vi "Dashboard Main.vi"() -> ()   [LabVIEW 2015]
uses:
  <vilib>/vision/Image Controls.llb/IMAQ Image.ctl
  <vilib>/Utility/miscctls.llb/LVRowAndColumnTypeDef.ctl
  <vilib>/event_ctls.llb/eventvkey.ctl
  <vilib>/Rock Robotics/WPI/Dashboard/WPI_DashboardLogging Global.vi
  <vilib>/Rock Robotics/Network Tables/NT Read Numeric Array.vi
  <vilib>/Rock Robotics/Network Tables/NT Read Boolean.vi
  <vilib>/Rock Robotics/Network Tables/NT Read Raw.vi
  <vilib>/Rock Robotics/Network Tables/NT Write Boolean.vi
  <vilib>/Utility/config.llb/Write Key (String).vi
  <vilib>/Utility/config.llb/Write Key (I32).vi
  <vilib>/Utility/config.llb/NI_LVConfig.lvlib
panel:
  in  "TCP":refnum<k5>
  in  "Rec Mode":enum32{"Stop", "Record", "Playback"}(radio)
  in  "Vision":u16(ring) items=["Camera Off", "USB Camera SW", "USB Camera HW", "IP Camera"]
  out "Camera IP":string
  out "Image Message":string="Timeout in Camera Communications"
  in  "Dashboard Tab":T1(tab)
  in  "CDF":bool
  in  "Position":i8
  in  "Power":i8(slide) scale=0.0..100.0
  in  "Select Auto":string(combo)
  out "NT Connection":bool
  in  "Camera Settings":T2={"Frame Rate"=30, "Compression"=30, "Size"=1} {"Frame Rate" scale=1.0..30.0; "Size" items=["640x480", "320x240", "160x120"]}
  out "MotorChart R":cluster{"Numeric":dbl, "Numeric":dbl}(graph)
  out "MotorChart L":T3(graph)
  out "MotorSliders R":cluster{"MotorSlide1":dbl, "MotorSlide2":dbl} {"MotorSlide2" scale=-1.0..1.0 scale format="%#_2e"; "MotorSlide1" scale=-1.0..1.0 scale format="%#_2e"}
  out "MotorSliders L":T4 {"MotorSlide4 2" scale=0.0..14.0 scale format="%#_2e"; "MotorSlide2" scale=-1.0..1.0 scale format="%#_2e"; "MotorSlide1" scale=-1.0..1.0 scale format="%#_2e"}
  out "JS1 Z":dbl(slide) scale=-1.0..1.0 scale format="%#_2e"
  out "JS1 Graph":cluster{"X":dbl, "Y":dbl}[](graph)
  out "JS1 Buttons":T5
  out "JS2 Z":dbl(slide) scale=-1.0..1.0 scale format="%#_2e"
  out "JS2 Graph":cluster{"X":dbl, "Y":dbl}[](graph)
  out "JS2 Buttons":T5
  out "Mode":T6(ring)=enum."Auto Disabled"
  in  "DB Camera Config":bool
  out "fps":dbl format="%#.1g"
  out "Mbps":dbl format="%#.1g"
  out "Mbps LED":bool
  in  "DB/String 9":string
  in  "DB/String 8":string
  in  "DB/String 7":string
  in  "DB/String 6":string
  in  "DB/String 5":string
  in  "DB/String 4":string
  in  "DB/String 3":string
  in  "DB/String 2":string
  in  "DB/String 1":string
  in  "DB/String 0":string
  in  "DB/Slider 0":dbl(slide) scale=0.0..5.0
  in  "DB/Slider 1":dbl(slide) scale=0.0..5.0
  in  "DB/Slider 2":dbl(slide) scale=0.0..5.0
  in  "DB/Slider 3":dbl(slide) scale=0.0..5.0
  out "DB/LED 3":bool
  out "DB/LED 2":bool
  out "DB/LED 1":bool
  out "DB/LED 0":bool
  in  "DB/Button 3":bool
  in  "DB/Button 2":bool
  in  "DB/Button 1":bool
  in  "DB/Button 0":bool caption="New Name"
  out "Masked Image":T7
  out "T3 Visible":bool
  out "T2 Visible":bool
  out "T1 Visible":bool
  out "Right":dbl(slide) scale=-1.0..1.0
  out "Left":dbl(slide) scale=-1.0..1.0
  out "T3 Y":dbl
  out "T3 X":dbl
  out "T2 Y":dbl
  out "T2 X":dbl
  out "TI Y":dbl
  out "T1 X":dbl
  out "T3 Dist":dbl
  out "T2 Dist":dbl
  out "T1 Dist":dbl
  out "Encoder 2 Dist":dbl
  out "Encoder 1 Dist":dbl
  out "Encoder 2 Dir":bool
  out "Encoder 1 Dir":bool
  in  "Test Slider":dbl(slide) scale=0.0..100.0 scale format="%#_3g"
  in  "On/Off":bool caption="Solenoid"
  in  "Test Name":u16(ring) items=["Select the test to run..."]
  in  "Test Tree":string(tree)
  in  "Motor":cluster{"Value":dbl, "Enable":bool} {"Value" scale=-1.0..1.0 scale format="%#_3g"}
  out "Progress":T8 {"Test Progress" scale=0.0..100.0}
  in  "Rev/Fwd":cluster{"Forward":bool, "Reverse":bool}
  in  "Test Ring":u16(ring) items=["Monochrome", "Color"]
  out "Cmd Status":string
  in  "Execute Command":bool
  in  "Command Params":string[][](table)
  in  "Command Selection":i32(listbox)
  in  "CheckList":i32(listbox)
  out "Tree":string(tree)
  out "Camera Image":T7(plugin-control)
  out "Background":bool
  # "Left"
  # "Front"
  # "Right"
  # "Battery"
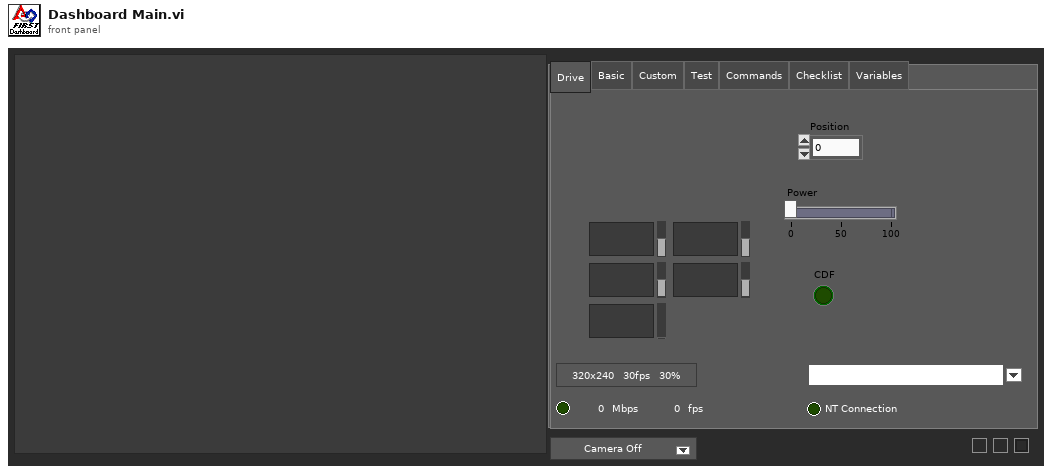
[diagram p1: front panel]
types:
  T1 = enum32{"Drive", "Basic", "Custom", "Test", "Commands", "Checklist", "Variables"}
  T2 = cluster{"Frame Rate":i32, "Compression":i32, "Size":u16}
  T3 = cluster{"Numeric":dbl, "Numeric":dbl, "Battery V":dbl}
  T4 = cluster{"MotorSlide1":dbl, "MotorSlide2":dbl, "MotorSlide4 2":dbl}
  T5 = cluster{bool, bool, bool, bool, bool, bool, bool, bool, bool, bool, bool, bool}
  T6 = enum8{"Tele-Op Disabled", "Tele-Op Enabled", "Auto Disabled", "Auto Enabled", "Test Disabled", "Test Enabled", "Disconnected", "No Code", "E-Stop"}
  T7 = typedef "IMAQ Image.ctl" = refnum<image>
  T8 = cluster{"Test Progress":u8, "Test Progress Text":string}
  T9 = cluster{"IDs":cluster{"RPC field ID":u16, "Unique ID":u16}, "String":string}
  T10 = enum32{"Drive", "Basic", "Custom", "Test", "Checklist", "Variables"}
  T11 = typedef "Image Type" = u32
  T12 = cluster{"Camera Image":refnum<vi>, "Dashboard Tab":refnum<vi>, "Background":refnum<vi>, "Vision":refnum<vi>, "Rec Mode":refnum<vi>, "Test Slider":refnum<vi>, "On/Off ":refnum<vi>, "Test Ring":refnum<vi>, "Rev/Fwd":refnum<vi>, "Test Name":refnum<vi>, "Motor":refnum<vi>, "Progress":refnum<vi>, "CheckList":refnum<vi>, "Tree":refnum<vi>, "Test Tree":refnum<vi>, "Command Params":refnum<vi>, "Command Selection":refnum<vi>, "Execute Command":refnum<vi>, "Cmd Status":refnum<vi>}
  T13 = cluster{"Error Strings":string, "Disable Counts":cluster{u16, u16}, "Rail Faults":cluster{u16, u16, u16}, "Robot IP":string, "DB Mode":u8, "Event Info":cluster{"Name":string, "Type":u8, "Number":u16, "Replay":u8}, "Camera Addr":string}
  T14 = cluster{"Storage":cluster{"Disk Free":u64, "RAM Block":u32, "RAM free":u32}, "CPU Utilization":cluster{"CPU % ISR":sgl, "CPU % Time Crit":sgl, "CPU % Timed Str":sgl, "CPU % High":sgl, "CPU % Above":sgl, "CPU % Normal":sgl, "CPU % Low":sgl}, "CAN":cluster{"% Bus Utilization":sgl, "Bus Off Cnt":u32, "TX_FIFO Full Cnt":u32, "Receive Error Cnt":u8, "Transmit Error Cnt":u8}, "HID":cluster{"HID Outputs":u32, "Rumble Low":u16, "Rumble High":u16}[]}
  T15 = cluster{"Status bits":cluster{"Test Mode":bool, "Autonomous":bool, "Enabled":bool, "Code Start":bool, "Brownout":bool, "Reserved 2":bool, "Reserved 3":bool, "E-Stop":bool}, "Code Trace":cluster{"Disabled":bool, "TeleOp":bool, "Auto":bool, "Test":bool}, "Controller Type":enum16{"unknown", "cRIO", "roboRio"}, "Code?":enum16{"unknown", "noCode", "code"}, "Battery V":dbl}
  T16 = cluster{"Control Bits":cluster{"TestMode":bool, "Autonomous":bool, "Enabled":bool, "FMS Present":bool, bool, bool, bool, "E-Stop":bool}, "Team Station ":u8, "Countdown":sgl, "Joystick Values":cluster{"Axes":dbl[], "Buttons":bool[], "POVs":i16[]}[]}
  T17 = cluster{"Axes":dbl[], "Buttons":bool[], "POVs":i16[]}[]
  T18 = cluster{"Axes":dbl[], "Buttons":bool[], "POVs":i16[]}
  T19 = cluster{"Buttons[0]":bool, "Buttons[1]":bool, "Buttons[2]":bool, "Buttons[3]":bool, "Buttons[4]":bool, "Buttons[5]":bool, "Buttons[6]":bool, "Buttons[7]":bool, "Buttons[8]":bool, "Buttons[9]":bool, "Buttons[10]":bool, "Buttons[11]":bool}
  T20 = typedef "NI_LVConfig.lvlib/Config Data RefNum.ctl" = refnum<k1>
  T21 = cluster{"Operation":enum16{"Update", "Clear"}, "Color Box":u32}[]
  T22 = typedef "eventvkey.ctl" = enum16{"ASCII", "Enter", "Return", "Shift", "Ctrl", "Alt", "Cmd", "Opt", "Caps", "NumLock", "Clear", "Break", "Up", "Down", "Left", "Right", "Insert", "Delete", "Home", "End", "PageUp", "PageDown", "Escape", "Help", "Pause", "ScrollLock", "F1", "F2", "F3", "F4", "F5", "F6", "F7", "F8", "F9", "F10", "F11", "F12", "F13", "F14", "F15", "F16", "F17", "F18", "F19", "F20", "F21", "F22", "F23", "F24", "Play", "VolumeUp", "VolumeDown", "Mute", "Two Byte Char"}
  T23 = cluster{"Image Size":bool, "Image Type":bool, "Pixel Value":bool, "ROI Information":bool, "Zoom Factor":bool}
  T24 = enum8{"Enabled", "Disabled", "Disabled and Grayed Out"}
  T25 = cluster{"Operation":enum16{"Update", "Clear"}, "Color Box":u32}
  T26 = typedef "LVRowAndColumnTypeDef.ctl" = cluster{"Row":i32, "Column":i32}
  T27 = cluster{"Shift":bool, "Ctrl":bool, "Alt":bool, "Cmd":bool, "Opt":bool}
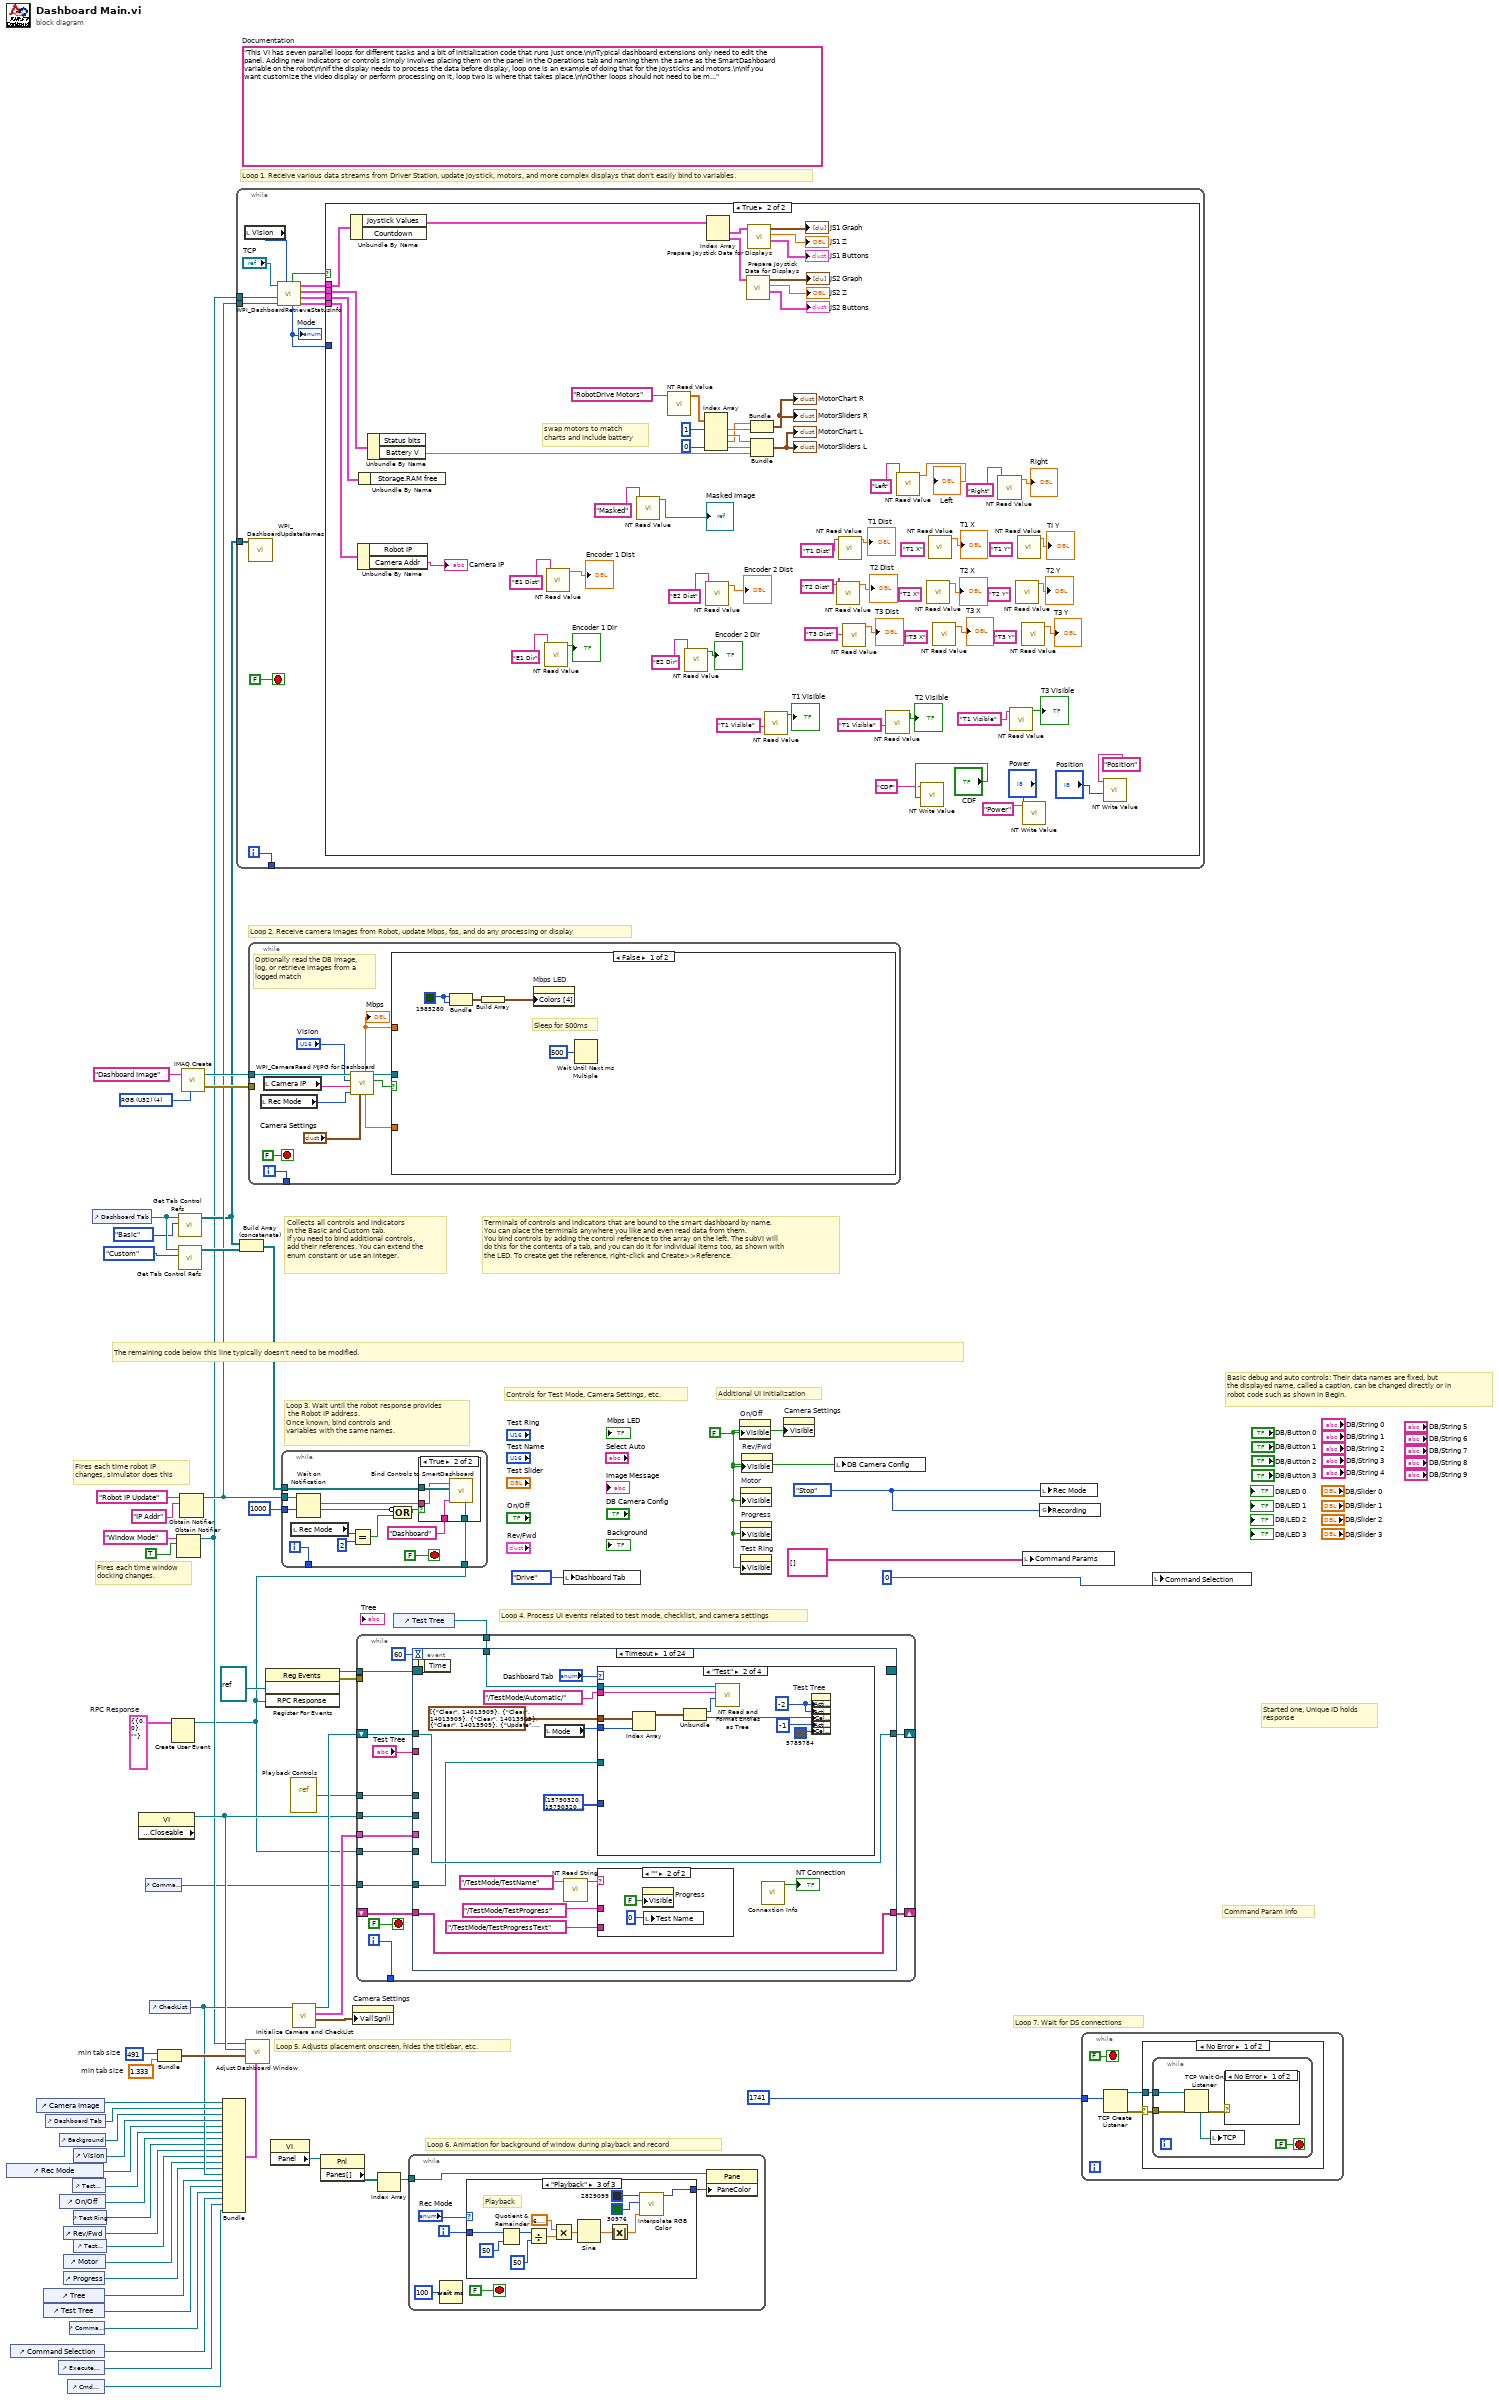
[diagram p0: block diagram]
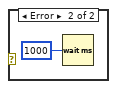
[diagram p2: hidden frame]
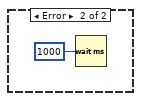
[diagram p3: hidden frame]
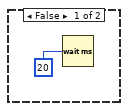
[diagram p4: hidden frame]
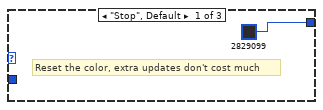
[diagram p5: hidden frame]
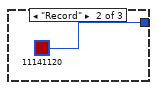
[diagram p6: hidden frame]
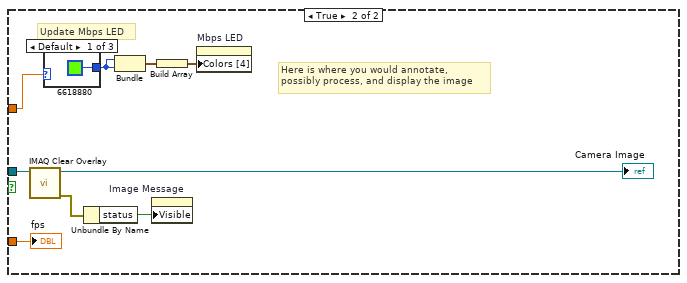
[diagram p8: hidden frame]
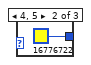
[diagram p9: hidden frame]
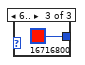
[diagram p10: hidden frame]
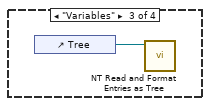
[diagram p12: hidden frame]
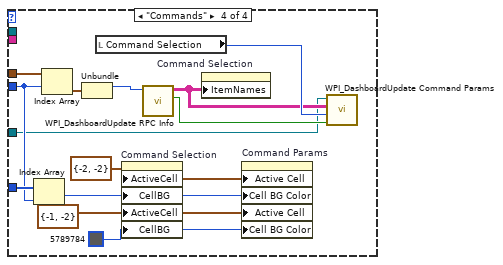
[diagram p13: hidden frame]
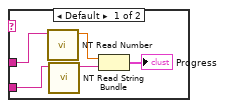
[diagram p14: hidden frame]
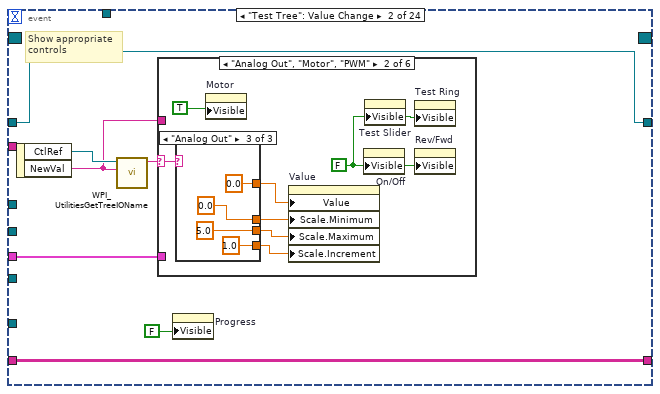
[diagram p15: hidden frame]
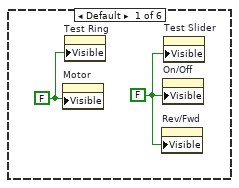
[diagram p16: hidden frame]
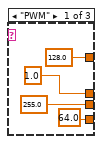
[diagram p17: hidden frame]
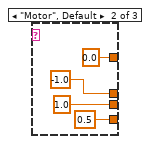
[diagram p18: hidden frame]
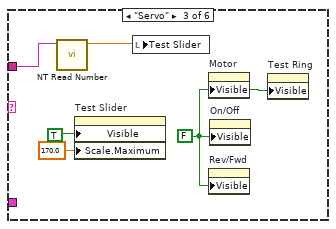
[diagram p19: hidden frame]
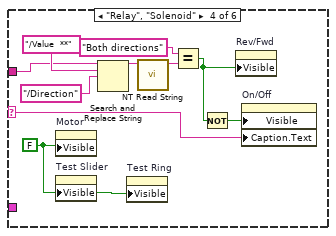
[diagram p20: hidden frame]
diagram:
  w7 = T9 {"IDs"={"RPC field ID"=0, "Unique ID"=0}, "String"=""}  # RPC Response
  w33 = 491  # min tab size
  w32 = 1.333  # min tab size
  w41 = enum32{"Stop", "Record", "Playback"}."Stop" ("Rec Mode")
  w15 = FALSE ("Visible")
  (unwired) "This VI has seven parallel loops for different tasks and a bit of initialization code that runs just once.\n\nTypical dashboard extensions only need to edit the panel. Adding new indicators or controls simply involves placing them on the panel in the Operations tab and naming them the same as the SmartDashboard variable on the robot\n\nIf the display needs to process the data before display, loop one is an example of doing that for the joysticks and motors.\n\nIf you want customize the video display or perform processing on it, loop two is where that takes place.\n\nOther loops should not need to be modified. They are pretty standard, and document the task they perform."  # Documentation
  w61 = T11 4 items=["Grayscale (U8)", "Grayscale (I16)", "Grayscale (SGL)", "Complex (CSG)", "RGB (U32)", "HSL (U32)", "RGB (U64)"] ("Image Type")
  # "Command Param Info"
  # "Started one, Unique ID holds\nresponse"
  # "Loop 7. Wait for DS connections"
  # "Basic debug and auto controls: Their data names are fixed, but\nthe displayed name, called a caption, can be changed directly or in\nrobot code such as shown in Begin."
  # "Controls for Test Mode, Camera Settings, etc."
  # "Additional UI Initialization"
  # "Loop 6. Animation for background of window during playback and record"
  # "Fires each time robot IP\nchanges, simulator does this"
  # "Fires each time window\ndocking changes."
  # "Collects all controls and indicators\nin the Basic and Custom tab.\nIf you need to bind additional controls,\nadd their references. You can extend the\nenum constant or use an integer."
  # "The remaining code below this line typically doesn't need to be modified."
  # "Loop 4. Process UI events related to test mode, checklist, and camera settings"
  # "Terminals of controls and indicators that are bound to the smart dashboard by name.\nYou can place the terminals anywhere you like and even read data from them.\nYou bind controls by adding the control reference to the array on the left. The subVI will\ndo this for the contents of a tab, and you can do it for individual items too, as shown with\nthe LED. To create get the reference, right-click and Create>>Reference."
  # "Loop 3. Wait until the robot response provides\n the Robot IP address.\nOnce known, bind controls and\nvariables with the same names."
  # "Loop 5. Adjusts placement onscreen, hides the titlebar, etc."
  # "Loop 1. Receive various data streams from Driver Station, update joystick, motors, and more complex displays that don't easily bind to variables."
  # "Loop 2. Receive camera images from Robot, update Mbps, fps, and do any processing or display"
  n1 = control-ref of="Rec Mode"() -> (w21:refnum<vi>)
  n2 = control-ref of="Command Selection"() -> (w6:refnum<vi>)
  n3 = control-ref of="Camera Image"() -> (w36:refnum<vi>)
  n4 = control-ref of="Tree"() -> (w25:refnum<vi>)
  n5 = control-ref of="Test Tree"() -> (w24:refnum<vi>)
  n6 = control-ref of="Dashboard Tab"() -> (w35:refnum<vi>)
  n7 = control-ref of="Execute Command"() -> (w8:refnum<vi>)
  n8 = control-ref of="Background"() -> (w30:refnum<vi>)
  n9 = control-ref of="On/Off"() -> (w19:refnum<vi>)
  n10 = control-ref of="Progress"() -> (w16:refnum<vi>)
  n11 = control-ref of="Rev/Fwd"() -> (w17:refnum<vi>)
  n12 = control-ref of="Motor"() -> (w22:refnum<vi>)
  n13 = control-ref of="Cmd Status"() -> (w2:refnum<vi>)
  n14 = control-ref of="Command Params"() -> (w9:refnum<vi>)
  n15 = control-ref of="Test Slider"() -> (w20:refnum<vi>)
  n16 = control-ref of="Vision"() -> (w34:refnum<vi>)
  n17 = control-ref of="Test Ring"() -> (w18:refnum<vi>)
  n18 = control-ref of="Test Name"() -> (w23:refnum<vi>)
  n19 = control-ref of="Dashboard Tab"() -> (w39:refnum<vi>)
  n20 = property class="VI" props=["Front Panel.Closeable"]() -> (reference out=w40:refnum<vi>)  [unwired: 2 in, 2 out]
  n21 = control-ref of="Command Params"() -> (w1:refnum<vi>)
  n22 = control-ref of="CheckList"() -> (w26:refnum<vi>)
  n23 = Bundle("min tab size"=w33, "min tab size"=w32) -> (w31:cluster{"min tab size":i32, "min tab size":dbl})  [unwired: 1 in]
  n24 = Create User Event(user event datatype=w7) -> (user event=w3:refnum<user-event>)  [unwired: 1 in, 1 out]
  n25 = Obtain Notifier(name (unnamed)="Window Mode", notification data type=TRUE) -> (notifier out=w12:refnum<notifier>)  [unwired: 2 in, 2 out]
  n26 = call <vilib>:"Get Tab Control Refs.vi"("Page Index"=T10."Basic" ("Dashboard Tab"), "TabControl in"=w39) -> ("ControlsOnPage"=w13:refnum<vi>[])  [unwired: 9 in]
  n27 = call <vilib>:"Get Tab Control Refs.vi"("Page Index"=T10."Custom" ("Dashboard Tab"), "TabControl in"=w39) -> ("ControlsOnPage"=w38:refnum<vi>[])  [unwired: 9 in]
  n28 = Obtain Notifier(name (unnamed)="Robot IP Update", notification data type="IP Addr" ("name (unnamed)")) -> (notifier out=w14:refnum<notifier>)  [unwired: 2 in, 2 out]
  n29 = call "IMAQ Create"("Image Name"="Dashboard Image", "Image Type"=w61) -> ("New Image"=w59:T7, "error out"=w58:errorcluster)  [unwired: 2 in, 1 out]
  n30 = Bundle("Camera Image"=w36, "Dashboard Tab"=w35, "Background"=w30, "Vision"=w34, "Rec Mode"=w21, "Test Slider"=w20, "On/Off"=w19, "Test Ring"=w18, "Rev/Fwd"=w17, "Test Name"=w23, "Motor"=w22, "Progress"=w16, "CheckList"=w26, "Tree"=w25, "Test Tree"=w24, "Command Params"=w9, "Command Selection"=w6, "Execute Command"=w8, "Cmd Status"=w2) -> (w27:T12)  [unwired: 1 in]
  n31 = while {
    tunnel: [w73] -> _
    tunnel: w14 -> [w67]
    tunnel: w13 -> [w66]
    tunnel: w12 -> [w62]
    i -> [w73]
    stop <- FALSE stop-if-true
    n32 = local read "Vision"() -> (w64:u16)
    n33 = call <vilib>:"WPI_DashboardUpdateNames.vi"("Controls on Tab"=w66) -> ()  [unwired: 11 in]
    n34 = call <vilib>:"WPI_DashboardRetrieveStatusInfo.vi"("Vision"=w64, "Binding Refnum"=w67, "Window Mode Notifier"=w62, "TCP Cnx"="TCP") -> ("Power and Errors"=w68:T13, "Robot Metrics"=w71:T14, "Status Info"=w72:T15, "Control Info"=w69:T16, "Robot Mode"=w65:T6, "Process?"=w70:bool)  [unwired: 2 in]
    "Mode" <- w65
    n35 = case shown="True" w70 {
      tunnel: w72 -> [_ w138]
      tunnel: w71 -> [_ w137]
      tunnel: w69 -> [_ w136]
      tunnel: w68 -> [_ w135]
      tunnel: w65 -> [_ _]
      frame False {
        n36 = Wait (ms)(milliseconds to wait=u32 20) -> ()  [unwired: 1 out]
      }
      frame True {
        (unwired) "T3 Y" ("Name")
        (unwired) "T3 X" ("Name")
        (unwired) "T2 Y" ("Name")
        (unwired) "T2 X" ("Name")
        (unwired) "T1 Y" ("Name")
        (unwired) "T1 X" ("Name")
        # "swap motors to match\ncharts and include battery"
        n37 = Unbundle By Name(w136) -> ("Joystick Values"=w125:T17)  [unwired: 1 out]
        n38 = Unbundle By Name(w135) -> ("Camera Addr"=→"Camera IP":string)  [unwired: 1 out]
        n39 = Unbundle By Name(w137) -> ()  [unwired: 1 out]
        n40 = Unbundle By Name(w138) -> ("Battery V"=w126:dbl)  [unwired: 1 out]
        n41 = call-poly <vilib>:"NT Read Value.vi"("Name"="E1 Dir") -> ("Boolean"=→"Encoder 1 Dir":bool)  [unwired: 9 in, 1 out]
        n42 = call-poly <vilib>:"NT Read Value.vi"("Name"="E1 Dist") -> ("Numeric"=→"Encoder 1 Dist":dbl)  [unwired: 9 in, 1 out]
        n43 = call-poly <vilib>:"NT Read Value.vi"("Name"="Masked") -> ("Raw"=→"Masked Image":string)  [unwired: 9 in, 1 out]
        n44 = call-poly <vilib>:"NT Read Value.vi"("Name"="RobotDrive Motors") -> ("Numeric Array"=w114:dbl[])  [unwired: 9 in, 1 out]
        n45 = call-poly <vilib>:"NT Read Value.vi"("Name"="E2 Dir") -> ("Boolean"=→"Encoder 2 Dir":bool)  [unwired: 9 in, 1 out]
        n46 = Index Array(array=w114, index #1=1, index #4=0) -> (element #1=w130:dbl, element #2=w131:dbl, element #3=w129:dbl, element #4=w134:dbl)  [unwired: 2 in]
        n47 = call-poly <vilib>:"NT Read Value.vi"("Name"="E2 Dist") -> ("Numeric"=→"Encoder 2 Dist":dbl)  [unwired: 9 in, 1 out]
        n48 = Index Array(array=w125) -> (element #1=w124:T18, element #2=w119:T18)  [unwired: 2 in]
        n49 = call "Prepare Joystick Data for Displays.vi"("Joystick Values"=w119) -> ("Buttons"=→"JS2 Buttons":T19, "Z Axis"=→"JS2 Z":dbl, "Cartesian Data"=→"JS2 Graph":cluster{"X axis":dbl, "X axis":dbl}[])  [unwired: 8 in]
        n50 = call "Prepare Joystick Data for Displays.vi"("Joystick Values"=w124) -> ("Buttons"=→"JS1 Buttons":T19, "Z Axis"=→"JS1 Z":dbl, "Cartesian Data"=→"JS1 Graph":cluster{"X axis":dbl, "X axis":dbl}[])  [unwired: 8 in]
        n51 = Bundle("Numeric"=w129, "Numeric"=w130) -> (→"MotorChart R" →"MotorSliders R":cluster{"Numeric":dbl, "Numeric":dbl})  [unwired: 1 in]
        n52 = Bundle("Numeric"=w131, "Numeric"=w134, "Battery V"=w126) -> (→"MotorChart L" →"MotorSliders L":T3)  [unwired: 1 in]
        n53 = call-poly <vilib>:"NT Read Value.vi"("Name"="T1 Visible") -> ("Boolean"=→"T1 Visible":bool)  [unwired: 9 in, 1 out]
        n54 = call-poly <vilib>:"NT Read Value.vi"("Name"="T2 Dist") -> ("Numeric"=→"T2 Dist":dbl)  [unwired: 9 in, 1 out]
        n55 = call-poly <vilib>:"NT Read Value.vi"("Name"="T1 Dist") -> ("Numeric"=→"T1 Dist":dbl)  [unwired: 9 in, 1 out]
        n56 = call-poly <vilib>:"NT Read Value.vi"("Name"="T3 Dist") -> ("Numeric"=→"T3 Dist":dbl)  [unwired: 9 in, 1 out]
        n57 = call-poly <vilib>:"NT Read Value.vi"("Name"="T1 Visible") -> ("Boolean"=→"T2 Visible":bool)  [unwired: 9 in, 1 out]
        n58 = call-poly <vilib>:"NT Read Value.vi"("Name"="Left") -> ("Numeric"=→"Left":dbl)  [unwired: 9 in, 1 out]
        n59 = call-poly <vilib>:"NT Write Value.vi"("Boolean"="CDF", "Name"="CDF") -> ()  [unwired: 9 in, 1 out]
        n60 = call-poly <vilib>:"NT Read Value.vi"() -> ("Numeric"=→"T2 X":dbl)  [unwired: 10 in, 1 out]
        n61 = call-poly <vilib>:"NT Read Value.vi"() -> ("Numeric"=→"T1 X":dbl)  [unwired: 10 in, 1 out]
        n62 = call-poly <vilib>:"NT Read Value.vi"() -> ("Numeric"=→"T3 X":dbl)  [unwired: 10 in, 1 out]
        n63 = call-poly <vilib>:"NT Read Value.vi"("Name"="Right") -> ("Numeric"=→"Right":dbl)  [unwired: 9 in, 1 out]
        n64 = call-poly <vilib>:"NT Read Value.vi"("Name"="T1 Visible") -> ("Boolean"=→"T3 Visible":bool)  [unwired: 9 in, 1 out]
        n65 = call-poly <vilib>:"NT Read Value.vi"() -> ("Numeric"=→"T2 Y":dbl)  [unwired: 10 in, 1 out]
        n66 = call-poly <vilib>:"NT Read Value.vi"() -> ("Numeric"=→"TI Y":dbl)  [unwired: 10 in, 1 out]
        n67 = call-poly <vilib>:"NT Read Value.vi"() -> ("Numeric"=→"T3 Y":dbl)  [unwired: 10 in, 1 out]
        n68 = call-poly <vilib>:"NT Write Value.vi"("Numeric"="Power", "Name"="Power") -> ()  [unwired: 9 in, 1 out]
        n69 = call-poly <vilib>:"NT Write Value.vi"("Numeric"="Position", "Name"="Position") -> ()  [unwired: 9 in, 1 out]
      }
    }
  }
  n70 = Build Array (concatenate)(w13, w38) -> (w37:refnum<vi>[])
  n71 = call "Adjust Dashboard Window.vi"("Sizing Refnums"=w27, "Size Constraints"=w31, "VI"=w40, "WIn Mode"=w12) -> ()  [unwired: 8 in]
  n72 = while {
    tunnel: w59 -> [w147]
    tunnel: w58 -> [_]
    tunnel: [w148] -> _
    i -> [w148]
    stop <- FALSE stop-if-true
    # "Optionally read the DB image,\nlog, or retrieve images from a\nlogged match"
    n73 = local read "Rec Mode"() -> (w142:enum32{"Stop", "Record", "Playback"})
    n74 = local read "Camera IP"() -> (w140:string)
    n75 = call <vilib>:"WPI_CameraRead MJPG for Dashboard.vi"("Camera Settings"="Camera Settings", "Rec Mode"=w142, "Camera IP"=w140, "Camera Mode"="Vision", "Refnum in"=w147) -> ("Active"=w145:bool, "Refnum out"=w146:T7, "FPS"=w144:dbl, "Bandwidth (Mbps)"=w139:dbl)  [unwired: 3 in]
    "Mbps" <- w139
    n76 = case shown="False" w145 {
      tunnel: w146 -> [_ w157]
      tunnel: w139 -> [_ w156]
      tunnel: w144 -> [_ w154]
      frame False {
        w150 = u32 1985280 ("Color Box")
        # "Sleep for 500ms"
        n77 = Bundle("Color Box"=w150, "Color Box"=w150) -> (w152:cluster{"Color Box":u32, "Color Box":u32})  [unwired: 1 out]
        n78 = Build Array(w152) -> (w151:cluster{"Color Box":u32, "Color Box":u32}[])
        n79 = property on="Mbps LED" class="Bool (strict)"("Colors [4]"=w151) -> ()  [unwired: 2 in, 2 out]
        n80 = Wait Until Next ms Multiple(millisecond multiple=u32 500) -> ()  [unwired: 1 out]
      }
      frame True {
        # "Here is where you would annotate,\npossibly process, and display the image"
        # "Update Mbps LED"
        n81 = call "IMAQ Clear Overlay"("Image"=w157) -> ("error out"=w161:errorcluster, "Image Out"=→"Camera Image":T7)  [unwired: 2 in, 7 out]
        n82 = case shown="Default" w156 {
          tunnel: [u32 6618880 ("Color Box") u32 16776722 ("Color Box") u32 16716800 ("Color Box")] -> w158
          frame Default {
          }
          frame 4, 5 {
          }
          frame 6.. {
          }
        }
        n83 = Unbundle By Name(w161) -> ("status"=w162:bool)
        n84 = Bundle("Color Box"=w158, "Color Box"=w158) -> (w160:cluster{"Color Box":u32, "Color Box":u32})  [unwired: 1 out]
        n85 = property on="Image Message" class="Str"("Visible"=w162) -> ()  [unwired: 2 in, 2 out]
        n86 = Build Array(w160) -> (w159:cluster{"Color Box":u32, "Color Box":u32}[])
        n87 = property on="Mbps LED" class="Bool (strict)"("Colors [4]"=w159) -> ()  [unwired: 2 in, 2 out]
        "fps" <- w154
      }
    }
  }
  n88 = register-events(refnum<vi> refnum, w3) -> (reference out=w45:refnum<event-registration>, error out=w44:errorcluster)  [unwired: 2 in]
  n89 = property class="VI"() -> ("Panel"=w48:refnum<vi>)  [unwired: 2 in, 2 out]
  n90 = while {
    tunnel: w37 -> [w178]
    tunnel: w14 -> [w176]
    tunnel: [w174] -> _
    tunnel: u32 1000 ("milliseconds to wait") -> [w173]
    tunnel: w3 -> [w166]
    i -> [w174]
    stop <- FALSE stop-if-true
    n91 = local read "Rec Mode"() -> (w169:enum32{"Stop", "Record", "Playback"})
    n92 = Wait on Notification(notifier=w176, timeout in ms (-1)=w173) -> (notification=w175:string, timed out?=w171:bool)  [unwired: 2 in, 2 out]
    n93 = Equal?(x=w169, y=u16 2 ("Rec Mode")) -> (x = y?=w170:bool)
    n94 = Compound Arithmetic op=OR(invert w171, w170) -> (w172:bool)
    n95 = case shown="True" w172 {
      tunnel: w178 -> [_ w182]
      tunnel: w175 -> [_ w181]
      tunnel: "Dashboard" -> [_ w180]
      tunnel: w166 -> [_ w179]
      frame False {
      }
      frame True {
        n96 = call <vilib>:"Bind Controls to SmartDashboard.vi"("RPC ref"=w179, "Client Name"=w180, "Bound Control Refs"=w182, "Server IP Address"=w181) -> ()  [unwired: 8 in]
      }
    }
  }
  n97 = vi-ref "Playback Controls.vi"() -> (w46:refnum<vi>)
  n98 = call "Initialize Camera and CheckList.vi"("ListBox in"=w26) -> ("Cluster"=w52:cluster{"value":i32, "value":i32, "index":i32}, "Array"=w53:cluster{string[]}[], "File Refnum"=w51:T20)  [unwired: 8 in]
  n99 = property class="Pnl"(reference=w48) -> ("Panes[]"=w49:refnum<vi>[])  [unwired: 1 in, 2 out]
  n100 = property on="Camera Settings" class="Clust (strict)"("Val(Sgnl)"=w52) -> ()  [unwired: 2 in, 2 out]
  n101 = Index Array(array=w49) -> (element=w47:refnum<vi>)  [unwired: 1 in]
  n102 = control-ref of="Test Tree"() -> (w50:refnum<vi>)
  n103 = while {
    tunnel: w53 -> [w194]
    shift-right: [w193] -> _
    shift-left: w51 -> [w192]
    tunnel: [w191] -> _
    tunnel: w50 -> [w190]
    tunnel: w46 -> [w189]
    tunnel: w45 -> [w188]
    tunnel: w44 -> [_]
    tunnel: w40 -> [w187]
    tunnel: w3 -> [w186]
    tunnel: w1 -> [w185]
    shift-right: [w184] -> _
    shift-left: _ -> [w183]
    i -> [w191]
    stop <- FALSE stop-if-true
    n104 = event shown="[0] Timeout" {
      selector: w188 -> [_ _ _ _ _ _ _ _ _ _ _ _ _ _ _ _ _ _ _ _ _ _ _ _]
      dyn-events: [_ _ _ _ _ _ _ _ _ _ _ _ _ _ _ _ _ _ w503 _ _ _ _ _] -> _
      timeout: u32 60 ("milliseconds to wait") -> [_ _ _ _ _ _ _ _ _ _ _ _ _ _ _ _ _ _ _ _ _ _ _ _]
      tunnel: w190 -> [w207 _ _ _ _ _ _ _ _ _ _ _ _ _ _ _ _ _ _ _ _ _ _ _]
      tunnel: "Test Tree" -> [_ _ _ _ _ _ _ _ _ _ _ _ _ w466 w475 w478 w483 w492 _ _ _ _ _ _]
      tunnel: w194 -> [_ w245 _ _ _ _ _ _ _ _ _ w428 w459 _ _ _ _ _ _ _ _ _ _ _]
      tunnel: [w204 w244 w348 w354 w364 w368 w374 w386 w394 w400 w413 w427 w452 w465 w473 w477 w482 w491 w505 w521 w523 w531 w542 w547] -> w193
      tunnel: w192 -> [w204 w244 w348 w354 w364 w368 w374 w386 w394 w400 w413 w426 w452 w465 w473 w477 w482 w491 w505 w521 w523 w531 w542 w547]
      tunnel: w189 -> [_ _ _ _ _ _ _ _ _ _ _ _ _ _ _ _ _ _ w506 _ w526 _ _ _]
      tunnel: w187 -> [_ _ _ _ _ _ _ _ _ _ _ _ _ _ _ _ _ _ w501 _ _ _ _ _]
      tunnel: w186 -> [_ _ _ _ _ _ _ _ _ _ _ _ _ _ _ _ _ _ w497 _ _ _ _ _]
      tunnel: w185 -> [w199 _ _ _ _ _ w372 _ _ _ _ _ _ _ _ _ _ _ _ _ _ _ _ _]
      tunnel: [w198 w243 w347 w353 w363 w369 w370 w380 w391 w399 w412 w425 w451 w464 w472 w476 w481 w490 w496 w519 w522 w527 w535 w548] -> w184
      tunnel: w183 -> [w198 w243 w347 w353 w363 w369 w370 _ _ w399 w412 w425 w451 w464 w472 w476 w481 w490 w496 w519 w522 w527 w535 w548]
      event Timeout {
        n105 = event-data() -> ()  [unwired: 1 in, 1 out]
        n106 = local read "Mode"() -> (w201:T6)
        n107 = call <vilib>:"NT Read String.vi"("Name"="/TestMode/TestName") -> ("String"=w210:string)  [unwired: 9 in, 1 out]
        n108 = case shown="\"Test\"" "Dashboard Tab" {
          tunnel: w207 -> [_ w221 _ _]
          tunnel: "/TestMode/Automatic/" ("Name Pattern") -> [_ w220 _ _]
          tunnel: T21 [{"Operation"=enum."Clear", "Color Box"=14013909}, {"Operation"=enum."Clear", "Color Box"=14013909}, {"Operation"=enum."Clear", "Color Box"=14013909}, {"Operation"=enum."Clear", "Color Box"=14013909}, {"Operation"=enum."Update", "Color Box"=14013909}, {"Operation"=enum."Update", "Color Box"=16777215}, {"Operation"=enum."Clear", "Color Box"=14013909}, {"Operation"=enum."Clear", "Color Box"=14013909}, {"Operation"=enum."Clear", "Color Box"=14013909}] -> [_ w213 _ w230]
          tunnel: w201 -> [_ w212 _ w229]
          tunnel: u32[] [15790320, 15790320, 15790320, 15790320, 16777215, 16777215, 15790320, 15790320, 15790320] -> [_ _ _ w235]
          tunnel: w199 -> [_ _ _ w223]
          frame "Custom", Default {
          }
          frame "Test" {
            w219 = -2 ("Active Item:Row Number")
            n109 = Index Array(array=w213, index=w212) -> (element=w214:T25)
            n110 = Unbundle(w214) -> ("Operation"=w215:enum16{"Update", "Clear"}, "Color Box"=w216:u32)
            n111 = call <vilib>:"NT Read and Format Entries as Tree.vi"("Operation"=w215, "Name Pattern"=w220, "Tree Refnum"=w221) -> ()  [unwired: 7 in, 2 out]
            n112 = property on="Test Tree" class="Tree (strict)"("Active Item Row Number"=w219, "ActiveColNum"=w219, "CellBG"=w216, "Active Item Row Number"=-1 ("Active Item:Row Number"), "CellBG"=u32 5789784 ("Color Box")) -> ()  [unwired: 2 in, 2 out]
          }
          frame "Variables" {
            n113 = control-ref of="Tree"() -> (w222:refnum<vi>)
            n114 = call <vilib>:"NT Read and Format Entries as Tree.vi"("Tree Refnum"=w222) -> ()  [unwired: 9 in, 2 out]
          }
          frame "Commands" {
            w231 = u32 5789784 ("Color Box")
            w232 = T26 {"Row"=-1, "Column"=-2} ("Active Cell:Active Cell")
            w234 = T26 {"Row"=-2, "Column"=-2} ("Active Cell:Active Cell")
            n115 = Index Array(array=w235, index=w229) -> (element=w233:u32)
            n116 = Index Array(array=w230, index=w229) -> (element=w228:T25)
            n117 = Unbundle(w228) -> ("Operation"=w227:enum16{"Update", "Clear"})  [unwired: 1 out]
            n118 = local read "Command Selection"() -> (w226:i32)
            n119 = property on="Command Selection" class="MCListbox (strict)"("ActiveCell"=w234, "CellBG"=w233, "ActiveCell"=w232, "CellBG"=w231) -> ()  [unwired: 2 in, 2 out]
            n120 = call <vilib>:"WPI_DashboardUpdate RPC Info.vi"("Operation"=w227) -> ("update"=w225:bool, "commands"=w224:string[][])  [unwired: 9 in]
            n121 = property on="Command Selection" class="MCListbox (strict)"("ItemNames"=w224) -> ()  [unwired: 2 in, 2 out]
            n122 = property on="Command Params" class="Tbl (strict)"("Active Cell"=w234, "Cell BG Color"=w233, "Active Cell"=w232, "Cell BG Color"=w231) -> ()  [unwired: 2 in, 2 out]
            n123 = call <vilib>:"WPI_DashboardUpdate Command Params.vi"("Update"=w225, "NewVal"=w226, "Commands"=w224, "Param Tbl"=w223) -> ()  [unwired: 7 in, 1 out]
          }
        }
        n124 = case shown="\"\"" w210 {
          tunnel: "/TestMode/TestProgress" ("Name") -> [w237 _]
          tunnel: "/TestMode/TestProgressText" ("Name") -> [w236 _]
          frame Default {
            n125 = call <vilib>:"NT Read Number.vi"("Name"=w237) -> ("Numeric"=w238:dbl)  [unwired: 9 in, 1 out]
            n126 = call <vilib>:"NT Read String.vi"("Name"=w236) -> ("String"=w239:string)  [unwired: 9 in, 1 out]
            n127 = Bundle("Numeric"=w238, "String"=w239) -> (→"Progress":cluster{"Numeric":dbl, "String":string})  [unwired: 1 in]
          }
          frame "" {
            n128 = property on="Progress" class="Clust (strict)"("Visible"=FALSE) -> ()  [unwired: 2 in, 2 out]
            n129 = local write "Test Name"(u16 0) -> ()
          }
        }
        n130 = call <vilib>:"Connextion Info.vi"() -> ("Connected"=→"NT Connection":bool)  [unwired: 10 in, 1 out]
      }
      event "Test Tree": Value Change {
        # "Show appropriate\ncontrols"
        n131 = event-data() -> ("CtlRef"=w248:refnum<vi>, "NewVal"=w246:string)  [unwired: 1 in]
        n132 = call <vilib>:"WPI_UtilitiesGetTreeIOName.vi"("NewVal"=w246, "TreeControl in"=w248) -> ("I/O Name"=w249:string)  [unwired: 9 in]
        n133 = case shown="\"Analog Out\", \"Motor\", \"PWM\"" w249 {
          selector: w249 -> [_ w256 _ w278 w287 _]
          tunnel: w246 -> [_ _ w275 w277 _ w294]
          tunnel: w245 -> [_ _ _ _ _ w293]
          frame Default {
            w251 = FALSE ("Visible")
            w250 = FALSE ("Visible")
            n134 = property on="Motor" class="Clust (strict)"("Visible"=w250) -> ()  [unwired: 2 in, 2 out]
            n135 = property on="Test Ring" class="Ring (strict)"("Visible"=w250) -> ()  [unwired: 2 in, 2 out]
            n136 = property on="Rev/Fwd" class="Clust (strict)"("Visible"=w251) -> ()  [unwired: 2 in, 2 out]
            n137 = property on="On/Off" class="Bool (strict)"("Visible"=w251) -> ()  [unwired: 2 in, 2 out]
            n138 = property on="Test Slider" class="Slide (strict)"("Visible"=w251) -> ()  [unwired: 2 in, 2 out]
          }
          frame "Analog Out", "Motor", "PWM" {
            w257 = FALSE ("Visible")
            n139 = case shown="\"Analog Out\"" w256 {
              tunnel: [1.0 ("Value") -1.0 ("Value") 0.0 ("Value")] -> w255
              tunnel: [255.0 ("Value") 1.0 ("Value") 5.0 ("Value")] -> w254
              tunnel: [128.0 ("Value") 0.0 ("Value") 0.0 ("Value")] -> w253
              tunnel: [64.0 ("Value") 0.5 ("Value") 1.0 ("Value")] -> w252
              frame "PWM" {
              }
              frame "Motor", Default {
              }
              frame "Analog Out" {
              }
            }
            n140 = property on="Motor" class="Clust (strict)"("Visible"=TRUE) -> ()  [unwired: 2 in, 2 out]
            n141 = property on="Value" class="Slide (strict)"("Value"=w253, "Scale.Minimum"=w255, "Scale.Maximum"=w254, "Scale.Increment"=w252) -> ()  [unwired: 2 in, 2 out]
            n142 = property on="On/Off" class="Bool (strict)"("Visible"=w257) -> ()  [unwired: 2 in, 2 out]
            n143 = property on="Test Slider" class="Slide (strict)"("Visible"=w257) -> ()  [unwired: 2 in, 2 out]
            n144 = property on="Test Ring" class="Ring (strict)"("Visible"=w257) -> ()  [unwired: 2 in, 2 out]
            n145 = property on="Rev/Fwd" class="Clust (strict)"("Visible"=w257) -> ()  [unwired: 2 in, 2 out]
          }
          frame "Servo" {
            w273 = FALSE ("Visible")
            n146 = call <vilib>:"NT Read Number.vi"("Name"=w275) -> ("Numeric"=w274:dbl)  [unwired: 9 in, 1 out]
            n147 = property on="Test Slider" class="Slide (strict)"("Visible"=TRUE, "Scale.Maximum"=170.0 ("Scale.Range:Maximum")) -> ()  [unwired: 2 in, 2 out]
            n148 = local write "Test Slider"(w274) -> ()
            n149 = property on="Motor" class="Clust (strict)"("Visible"=w273) -> ()  [unwired: 2 in, 2 out]
            n150 = property on="Rev/Fwd" class="Clust (strict)"("Visible"=w273) -> ()  [unwired: 2 in, 2 out]
            n151 = property on="On/Off" class="Bool (strict)"("Visible"=w273) -> ()  [unwired: 2 in, 2 out]
            n152 = property on="Test Ring" class="Ring (strict)"("Visible"=w273) -> ()  [unwired: 2 in, 2 out]
          }
          frame "Relay", "Solenoid" {
            w276 = FALSE ("Visible")
            n153 = property on="Motor" class="Clust (strict)"("Visible"=w276) -> ()  [unwired: 2 in, 2 out]
            n154 = property on="Test Slider" class="Slide (strict)"("Visible"=w276) -> ()  [unwired: 2 in, 2 out]
            n155 = Search and Replace String(input string=w277, search string="/Value  **", replace string="/Direction") -> (result string=w283:string)  [unwired: 5 in, 3 out]
            n156 = property on="Test Ring" class="Ring (strict)"("Visible"=w276) -> ()  [unwired: 2 in, 2 out]
            n157 = call <vilib>:"NT Read String.vi"("Name"=w283) -> ("String"=w281:string)  [unwired: 9 in, 1 out]
            n158 = Equal?(x="Both directions", y=w281) -> (x = y?=w279:bool)
            n159 = Not(x=w279) -> (.not. x?=w280:bool)
            n160 = property on="Rev/Fwd" class="Clust (strict)"("Visible"=w279) -> ()  [unwired: 2 in, 2 out]
            n161 = property on="On/Off" class="Bool (strict)"("Visible"=w280, "Caption.Text"=w278) -> ()  [unwired: 2 in, 2 out]
          }
          frame "Compressor", "Digital Out" {
            w286 = FALSE ("Visible")
            # "Get direction and finish"
            n162 = property on="Motor" class="Clust (strict)"("Visible"=w286) -> ()  [unwired: 2 in, 2 out]
            n163 = property on="Test Slider" class="Slide (strict)"("Visible"=w286) -> ()  [unwired: 2 in, 2 out]
            n164 = property on="Test Ring" class="Ring (strict)"("Visible"=w286) -> ()  [unwired: 2 in, 2 out]
            n165 = property on="On/Off" class="Bool (strict)"("Visible"=TRUE, "Caption.Text"=w287) -> ()  [unwired: 2 in, 2 out]
            n166 = property on="Rev/Fwd" class="Clust (strict)"("Visible"=FALSE) -> ()  [unwired: 2 in, 2 out]
          }
          frame "Camera" {
            n167 = call <vilib>:"Get Last Path Segment.vi"("String in"=w294) -> ("String out"=w295:string)  [unwired: 10 in]
            n168 = property on="On/Off" class="Bool (strict)"("Visible"=FALSE) -> ()  [unwired: 2 in, 2 out]
            n169 = property on="Motor" class="Clust (strict)"("Visible"=FALSE) -> ()  [unwired: 2 in, 2 out]
            n170 = property on="Rev/Fwd" class="Clust (strict)"("Visible"=FALSE) -> ()  [unwired: 2 in, 2 out]
            n171 = case shown="\"White Balance  **\"" w295 {
              tunnel: w294 -> [w301 w310 w319 w328 w337 _ w343]
              tunnel: w293 -> [w299 w307 w316 w325 w334 _ _]
              frame "Size  **" {
                n172 = Index Array(array=w299) -> (element=w298:cluster{string[]})  [unwired: 1 in]
                n173 = call <vilib>:"NT Read String.vi"("Name"=w301) -> ("String"=w300:string)  [unwired: 9 in, 1 out]
                n174 = Unbundle(w298) -> (w296:string[])
                n175 = Match First String(2:w296, 3:w300) -> (0:w297:i32)  [unwired: 1 out]
                n176 = property on="Test Ring" class="Ring (strict)"("Value"=w297, "Strings []"=w296) -> ()  [unwired: 2 in, 2 out]
                n177 = property on="Test Ring" class="Ring (strict)"("Visible"=TRUE) -> ()  [unwired: 2 in, 2 out]
                n178 = property on="Test Slider" class="Slide (strict)"("Visible"=FALSE) -> ()  [unwired: 2 in, 2 out]
              }
              frame "White Balance  **" {
                n179 = Index Array(array=w307, index=1) -> (element=w308:cluster{string[]})
                n180 = call <vilib>:"NT Read String.vi"("Name"=w310) -> ("String"=w309:string)  [unwired: 9 in, 1 out]
                n181 = Unbundle(w308) -> (w305:string[])
                n182 = Match First String(2:w305, 3:w309) -> (0:w304:i32)  [unwired: 1 out]
                n183 = property on="Test Ring" class="Ring (strict)"("Value"=w304, "Strings []"=w305) -> ()  [unwired: 2 in, 2 out]
                n184 = property on="Test Ring" class="Ring (strict)"("Visible"=TRUE) -> ()  [unwired: 2 in, 2 out]
                n185 = property on="Test Slider" class="Slide (strict)"("Visible"=FALSE) -> ()  [unwired: 2 in, 2 out]
              }
              frame "Exposure  **" {
                n186 = Index Array(array=w316, index=2) -> (element=w317:cluster{string[]})
                n187 = call <vilib>:"NT Read String.vi"("Name"=w319) -> ("String"=w318:string)  [unwired: 9 in, 1 out]
                n188 = Unbundle(w317) -> (w313:string[])
                n189 = Match First String(2:w313, 3:w318) -> (0:w314:i32)  [unwired: 1 out]
                n190 = property on="Test Ring" class="Ring (strict)"("Value"=w314, "Strings []"=w313) -> ()  [unwired: 2 in, 2 out]
                n191 = property on="Test Ring" class="Ring (strict)"("Visible"=TRUE) -> ()  [unwired: 2 in, 2 out]
                n192 = property on="Test Slider" class="Slide (strict)"("Visible"=FALSE) -> ()  [unwired: 2 in, 2 out]
              }
              frame "Exposure Priority  **" {
                n193 = Index Array(array=w325, index=3) -> (element=w326:cluster{string[]})
                n194 = call <vilib>:"NT Read String.vi"("Name"=w328) -> ("String"=w327:string)  [unwired: 9 in, 1 out]
                n195 = Unbundle(w326) -> (w322:string[])
                n196 = Match First String(2:w322, 3:w327) -> (0:w323:i32)  [unwired: 1 out]
                n197 = property on="Test Ring" class="Ring (strict)"("Value"=w323, "Strings []"=w322) -> ()  [unwired: 2 in, 2 out]
                n198 = property on="Test Ring" class="Ring (strict)"("Visible"=TRUE) -> ()  [unwired: 2 in, 2 out]
                n199 = property on="Test Slider" class="Slide (strict)"("Visible"=FALSE) -> ()  [unwired: 2 in, 2 out]
              }
              frame "Color Enable  **" {
                n200 = Index Array(array=w334, index=4) -> (element=w335:cluster{string[]})
                n201 = call <vilib>:"NT Read String.vi"("Name"=w337) -> ("String"=w336:string)  [unwired: 9 in, 1 out]
                n202 = Unbundle(w335) -> (w331:string[])
                n203 = Match First String(2:w331, 3:w336) -> (0:w332:i32)  [unwired: 1 out]
                n204 = property on="Test Ring" class="Ring (strict)"("Value"=w332, "Strings []"=w331) -> ()  [unwired: 2 in, 2 out]
                n205 = property on="Test Ring" class="Ring (strict)"("Visible"=TRUE) -> ()  [unwired: 2 in, 2 out]
                n206 = property on="Test Slider" class="Slide (strict)"("Visible"=FALSE) -> ()  [unwired: 2 in, 2 out]
              }
              frame Default {
                n207 = property on="Test Ring" class="Ring (strict)"("Visible"=FALSE) -> ()  [unwired: 2 in, 2 out]
                n208 = property on="Test Slider" class="Slide (strict)"("Visible"=FALSE) -> ()  [unwired: 2 in, 2 out]
              }
              frame "Brightness  **", "Color Level  **", "Compression  **", "FPS  **", "Sharpness  **" {
                n209 = call <vilib>:"NT Read Number.vi"("Name"=w343) -> ("Numeric"=w342:dbl)  [unwired: 9 in, 1 out]
                n210 = local write "Test Slider"(w342) -> ()
                n211 = property on="Test Slider" class="Slide (strict)"("Visible"=TRUE, "Scale.Maximum"=100.0 ("Scale.Range:Maximum")) -> ()  [unwired: 2 in, 2 out]
                n212 = property on="Test Ring" class="Ring (strict)"("Visible"=FALSE) -> ()  [unwired: 2 in, 2 out]
              }
            }
          }
        }
        n213 = property on="Progress" class="Clust (strict)"("Visible"=FALSE) -> ()  [unwired: 2 in, 2 out]
      }
      event "Test Name": Mouse Enter {
        # "Populate the ring with the list of tests"
        n214 = event-data() -> ()  [unwired: 1 in, 1 out]
        n215 = call <vilib>:"NT Read String Array.vi"("Name"="/TestMode/TestList") -> ("String Array"=w352:string[])  [unwired: 9 in, 1 out]
        n216 = Build Array (concatenate)("Select the test to run...", w352) -> (w351:string[])
        n217 = property on="Test Name" class="Ring (strict)"("Strings []"=w351) -> ()  [unwired: 2 in, 2 out]
      }
      event "Test Name": Value Change {
        w355 = FALSE ("Visible")
        # "Tell the robot the test name to run"
        n218 = event-data() -> ("NewVal"=w359:u16)  [unwired: 1 in]
        n219 = property on="Test Name" class="Ring (strict)"() -> ("Strings []"=w360:string[])  [unwired: 2 in, 2 out]
        n220 = local write "Progress"(T8 {"Test Progress"=0, "Test Progress Text"=""} ("Progress")) -> ()
        n221 = Index Array(array=w360, index=w359) -> (element=w358:string)
        n222 = call <vilib>:"NT Write String.vi"("String"=w358, "Name"="/TestMode/TestName") -> ()  [unwired: 9 in, 1 out]
        n223 = property on="Progress" class="Clust (strict)"("Visible"=TRUE) -> ()  [unwired: 2 in, 2 out]
        n224 = property on="Motor" class="Clust (strict)"("Visible"=w355) -> ()  [unwired: 2 in, 2 out]
        n225 = property on="Test Slider" class="Slide (strict)"("Visible"=w355) -> ()  [unwired: 2 in, 2 out]
        n226 = property on="On/Off" class="Bool (strict)"("Visible"=w355) -> ()  [unwired: 2 in, 2 out]
        n227 = property on="Rev/Fwd" class="Clust (strict)"("Visible"=w355) -> ()  [unwired: 2 in, 2 out]
        n228 = property on="Test Ring" class="Ring (strict)"("Visible"=w355) -> ()  [unwired: 2 in, 2 out]
      }
      event "Select Auto": Mouse Enter {
        # "Populate the combo box with the list of autonomous options"
        n229 = event-data() -> ()  [unwired: 1 in, 1 out]
        n230 = call <vilib>:"NT Read String Array.vi"("Name"="Auto List") -> ("String Array"=w362:string[])  [unwired: 9 in, 1 out]
        n231 = property on="Select Auto" class="CmbBox"("Strings[]"=w362) -> ()  [unwired: 2 in, 2 out]
      }
      event "Select Auto": Value Change {
        # "User modified the Auto Selection. Write to NT variable so robot knows."
        n232 = event-data() -> ("NewVal"=w366:string)  [unwired: 1 in]
        n233 = call <vilib>:"NT Write String.vi"("String"=w366, "Name"="Auto Selector") -> ()  [unwired: 9 in, 1 out]
      }
      event "Command Selection": Value Change {
        # "Get the params and show in table"
        n234 = event-data() -> ("NewVal"=w373:i32)  [unwired: 1 in]
        n235 = property on="Command Selection" class="MCListbox (strict)"() -> ("ItemNames"=w371:string[][])  [unwired: 2 in, 2 out]
        n236 = call <vilib>:"WPI_DashboardUpdate Command Params.vi"("NewVal"=w373, "Commands"=w371, "Param Tbl"=w372) -> ()  [unwired: 8 in, 1 out]
      }
      event "Execute Command": Value Change {
        # "Started one, Unique ID holds\nresponse"
        n237 = event-data() -> ()  [unwired: 1 in, 1 out]
        n238 = property on="Command Selection" class="MCListbox (strict)"() -> ("ItemNames"=w385:string[][])  [unwired: 2 in, 2 out]
        n239 = Index Array(array=w385, index (row)="Command Selection", index (col)=0) -> (element=w383:string)
        n240 = call <vilib>:"Invoke Commands.vi"("Command Params"="Command Params", "Function Name"=w383) -> ("Params"=w379:u8, "Started"=w378:bool)  [unwired: 7 in, 1 out]
        n241 = Array Subset(array="Command Params", length (row)=w379) -> (w380:string[][])  [unwired: 3 in]
        n242 = Select(t="Executing" ("Cmd Status"), s=w378, f="" ("Cmd Status")) -> (s? t:f=→"Cmd Status":string)
      }
      event "Command Selection": Double Click {
        n243 = event-data() -> ("Row"=w395:i32)  [unwired: 1 in]
        n244 = property on="Command Selection" class="MCListbox (strict)"() -> ("ItemNames"=w398:string[][])  [unwired: 2 in, 2 out]
        n245 = local read "Command Params"() -> (w393:string[][])
        n246 = Index Array(array=w398, index (row)=w395, index (col)=0) -> (element=w396:string)
        n247 = call <vilib>:"Invoke Commands.vi"("Command Params"=w393, "Function Name"=w396) -> ("Params"=w392:u8, "Started"=w387:bool)  [unwired: 7 in, 1 out]
        n248 = Array Subset(array=w393, length (row)=w392) -> (w391:string[][])  [unwired: 3 in]
        n249 = Select(t="Executing" ("Cmd Status"), s=w387, f="" ("Cmd Status")) -> (s? t:f=w388:string)
        n250 = local write "Cmd Status"(w388) -> ()
      }
      event "CheckList": Double Click {
        # "Shift clears all"
        # "Update symbols on the listbox"
        n251 = event-data() -> ("PlatMods.Shift"=w401:bool, "Row"=w403:i32)  [unwired: 1 in]
        n252 = case shown="True" w401 {
          tunnel: w403 -> [w407 _]
          tunnel: 1 -> [w406 _]
          frame False {
            n253 = property on="CheckList" class="LstBox (strict)"() -> ("Item Symbols"=w405:i32[])  [unwired: 2 in, 2 out]
            n254 = Replace Array Subset(array=w405, new element=w406, index=w407) -> (w404:i32[])
            n255 = property on="CheckList" class="LstBox (strict)"("Item Symbols"=w404) -> ()  [unwired: 2 in, 2 out]
          }
          frame True {
            w408 = 0 ("Top Row")
            n256 = property on="CheckList" class="LstBox (strict)"() -> ("Number of Rows"=w410:u32)  [unwired: 2 in, 2 out]
            n257 = Initialize Array(0, w410) -> (w409:i32[])
            n258 = property on="CheckList" class="LstBox (strict)"("Top Row"=w408, "Value"=w408, "Item Symbols"=w409) -> ()  [unwired: 2 in, 2 out]
          }
        }
      }
      event "CheckList": Key Down {
        # "Update symbols on the listbox\nLeft and right keys check and uncheck"
        n259 = event-data() -> ("VKey"=w415:T22)  [unwired: 1 in]
        n260 = case shown="\"Left\", \"Right\"" w415 {
          selector: w415 -> [w420 _]
          tunnel: eventvkey."Left" ("VKey") -> [w418 _]
          frame "Left", "Right" {
            n261 = Equal?(x=w418, y=w420) -> (x = y?=w419:bool)
            n262 = Select(t=0, s=w419, f=1) -> (s? t:f=w421:i32)
            n263 = property on="CheckList" class="LstBox (strict)"() -> ("Item Symbols"=w424:i32[])  [unwired: 2 in, 2 out]
            n264 = Replace Array Subset(array=w424, new element=w421, index="CheckList") -> (w423:i32[])
            n265 = property on="CheckList" class="LstBox (strict)"("Item Symbols"=w423) -> ()  [unwired: 2 in, 2 out]
          }
          frame Default {
          }
        }
      }
      event "DB Camera Config": Value Change {
        # "Show or hide the cluster of controls, store in ini file"
        n266 = event-data() -> ("NewVal"=w429:bool)  [unwired: 1 in]
        n267 = case shown="False" w429 {
          tunnel: w428 -> [w438 _]
          tunnel: [w431 w449] -> w427
          tunnel: w426 -> [w430 w449]
          frame False {
            w445 = "Camera"
            w448 = FALSE ("Visible")
            n268 = local read "Camera Settings"() -> (w437:T2)
            n269 = Index Array(array=w438) -> (element=w441:cluster{string[]})  [unwired: 1 in]
            n270 = Unbundle(w437) -> ("Frame Rate"=w436:i32, "Compression"=w435:i32, "Size"=w439:u16)
            n271 = Unbundle(w441) -> (w440:string[])
            n272 = Index Array(array=w440, index=w439) -> (element=w434:string)
            n273 = call-poly <vilib>:"Write Key.vi"("section"=w445, "value"=w434, "key"="Size", "refnum"=w430) -> ("refnum out"=w447:T20)  [unwired: 2 in, 5 out]
            n274 = call-poly <vilib>:"Write Key.vi"("section"=w445, "value"=w436, "key"="FrameRate", "refnum"=w447) -> ("refnum out"=w446:T20)  [unwired: 1 in, 6 out]
            n275 = property on="Camera Settings" class="Clust (strict)"("Visible"=w448) -> ()  [unwired: 2 in, 2 out]
            n276 = local write "DB Camera Config"(w448) -> ()
            n277 = call-poly <vilib>:"Write Key.vi"("section"=w445, "value"=w435, "key"="Compression", "refnum"=w446) -> ("refnum out"=w432:T20)  [unwired: 1 in, 6 out]
            n278 = call <vilib>:"Close Config Data.vi"("refnum"=w432) -> ("file path"=w433:path)  [unwired: 2 in, 8 out]
            n279 = call <vilib>:"Open Config Data.vi"("configuration file path"=w433) -> ("refnum"=w431:T20)  [unwired: 8 in, 2 out]
          }
          frame True {
            n280 = property on="Camera Settings" class="Clust (strict)"("Visible"=TRUE) -> ()  [unwired: 2 in, 2 out]
          }
        }
      }
      event "Camera Settings": Value Change {
        # "Update summary string when any elements of DB camera change"
        n281 = event-data() -> ("NewVal"=w463:T2)  [unwired: 1 in]
        n282 = Index Array(array=w459) -> (element=w458:cluster{string[]})  [unwired: 1 in]
        n283 = Unbundle(w463) -> ("Frame Rate"=w454:i32, "Compression"=w453:i32, "Size"=w456:u16)
        n284 = Unbundle(w458) -> (w457:string[])
        n285 = Index Array(array=w457, index=w456) -> (element=w455:string)
        n286 = Format Into String(format string="%s   %dfps   %d%%", w455, w454, w453) -> (resulting string=w460:string)  [unwired: 2 in, 1 out]
        n287 = Build Array(w460) -> (w461:string[])
        n288 = property on="DB Camera Config" class="Bool (strict)"("Strings [4]"=w461) -> ()  [unwired: 2 in, 2 out]
      }
      event "Motor.Enable": Value Change {
        # "When the test mode otor enable helper is set, update that\ntree row item's value"
        n289 = event-data() -> ("NewVal"=w470:bool)  [unwired: 1 in]
        n290 = Unbundle("Motor") -> ("Value"=w469:dbl)  [unwired: 1 out]
        n291 = Select(t=w469, s=w470, f=0.0) -> (s? t:f=w467:dbl)
        n292 = call <vilib>:"NT Write Number.vi"("Numeric"=w467, "Name"=w466) -> ()  [unwired: 9 in, 1 out]
      }
      event "Test Slider": Value Change {
        # "When the test mode slider helper is set, update that\ntree row item's value"
        n293 = event-data() -> ("NewVal"=w474:dbl)  [unwired: 1 in]
        n294 = call <vilib>:"NT Write Number.vi"("Numeric"=w474, "Name"=w475) -> ()  [unwired: 9 in, 1 out]
      }
      event "On/Off": Value Change {
        # "When the test mode on/off helper value is set, update that\ntree row item's value"
        n295 = event-data() -> ("NewVal"=w480:bool)  [unwired: 1 in]
        n296 = Boolean To (0,1)(Boolean=w480) -> (0, 1=w479:i16)
        n297 = call <vilib>:"NT Write Number.vi"("Numeric"=w479, "Name"=w478) -> ()  [unwired: 9 in, 1 out]
      }
      event "Rev/Fwd": Value Change {
        # "When the test mode helper value for relays is set, update that\ntree row item's value"
        n298 = event-data() -> ("NewVal.Forward"=w489:bool, "NewVal.Reverse"=w488:bool)  [unwired: 1 in]
        n299 = Boolean To (0,1)(Boolean=w489) -> (0, 1=w485:i16)
        n300 = Boolean To (0,1)(Boolean=w488) -> (0, 1=w487:i16)
        n301 = Negate(x=w487) -> (-x=w486:i16)
        n302 = Add(x=w485, y=w486) -> (x+y=w484:i16)
        n303 = call <vilib>:"NT Write Number.vi"("Numeric"=w484, "Name"=w483) -> ()  [unwired: 9 in, 1 out]
      }
      event "Test Ring": Value Change {
        # "When a test mode helper value is selected from the ring,\nset the tree item's variable to the string value"
        n304 = event-data() -> ("NewVal"=w494:u16)  [unwired: 1 in]
        n305 = property on="Test Ring" class="Ring (strict)"() -> ("Strings []"=w495:string[])  [unwired: 2 in, 2 out]
        n306 = Index Array(array=w495, index=w494) -> (element=w493:string)
        n307 = call <vilib>:"NT Write String.vi"("String"=w493, "Name"=w492) -> ()  [unwired: 9 in, 1 out]
      }
      event "Rec Mode": Value Change {
        # "Update globals for recording mode and path to read log from.\nClear when logging and let NetworkTables set path for vision to\nuse."
        n308 = event-data() -> ("NewVal"=w507:enum32{"Stop", "Record", "Playback"})  [unwired: 1 in]
        n309 = global write "WPI_DashboardLogging Global.vi" "Logging Filename"(path "") -> ()
        n310 = global write "WPI_DashboardLogging Global.vi" "Recording"(w507) -> ()
        n311 = case shown="\"Playback\"" w507 {
          tunnel: w506 -> [_ w509 w518]
          tunnel: [_ _ w517] -> w503
          tunnel: [_ _ w516] -> _
          tunnel: w501 -> [_ _ w514]
          tunnel: cluster{i32, i32} {-250, 170} -> [_ _ w513]
          tunnel: [_ _ T23 {"Image Size"=TRUE, "Image Type"=TRUE, "Pixel Value"=TRUE, "ROI Information"=TRUE, "Zoom Factor"=FALSE} ("Image Information Shown:All Elements")] -> w499
          tunnel: [_ _ TRUE ("Zoom Factor")] -> w498
          tunnel: w497 -> [_ _ w510]
          frame Default {
          }
          frame "Stop", "Record" {
            # "Place Window too"
            n312 = invoke class="VI" method="FP.Close"(reference=w509) -> (reference out=w508:refnum<vi>)  [unwired: 2 in, 2 out]
            n313 = invoke class="VI" method="Abort VI"(reference=w508) -> ()  [unwired: 2 in, 3 out]
          }
          frame "Playback" {
            n314 = call "Open Playback Panel.vi"("Offset"=w513, "DB VI Ref"=w514, "Playback in"=w518) -> ("Playback out"=w515:refnum<vi>)  [unwired: 8 in]
            n315 = register-events(w515, w510) -> (reference out=w517:refnum<event-registration>, error out=w516:errorcluster)  [unwired: 2 in]
          }
        }
        n316 = property on="Camera Image" class="ImageControl"("Image Information Shown"=w499, "Image Information Visible"=w498) -> ()  [unwired: 2 in, 2 out]
        n317 = call <vilib>:"WPI_DashboardNT Log FieldName Cache.vi"("Operation"=enum16{"Lookup/Add", "Index", "Clear"}."Clear") -> ()  [unwired: 8 in, 3 out]
      }
      event Panel Close {
        w520 = enum32{"Stop", "Record", "Playback"}."Stop" ("Rec Mode")
        # "Playback window has been closed, abort"
        n318 = event-data() -> ()  [unwired: 1 in, 4 out]
        n319 = local write "Rec Mode"(w520) -> ()
        n320 = global write "WPI_DashboardLogging Global.vi" "Recording"(w520) -> ()
      }
      event Panel Close {
        # "Abort playback window and ourself"
        n321 = event-data() -> ()  [unwired: 1 in, 4 out]
        n322 = invoke class="VI" method="FP.Close"(reference=w526) -> (reference out=w525:refnum<vi>)  [unwired: 2 in, 2 out]
        n323 = invoke class="VI" method="Abort VI"(reference=w525) -> (error out=w524:errorcluster)  [unwired: 2 in, 2 out]
        n324 = invoke class="VI" method="Abort VI"(error in=w524) -> ()  [unwired: 2 in, 3 out]
      }
      event User Event {
        n325 = event-data() -> ("IDs"=w534:cluster{"RPC field ID":u16, "Unique ID":u16}, "String"=w533:string)  [unwired: 1 in]
        n326 = Bundle("IDs"=w534, "String"=w533) -> (w532:T9)  [unwired: 1 in]
        n327 = call <vilib>:"Retrieve RPC Response.vi"("RPC Response"=w532) -> ("Output"=w529:string[][])  [unwired: 10 in]
        n328 = Build Array (concatenate)(w527, w529) -> (w528:string[][])
        n329 = local write "Command Params"(w528) -> ()
        n330 = local write "Cmd Status"("" ("Cmd Status")) -> ()
      }
      event "Vision": Value Change {
        # "Enable/Disable Compression slider.\nHW USB is hard-coded into the camera"
        n331 = event-data() -> ("NewVal"=w541:u16)  [unwired: 1 in]
        n332 = Equal?(x=w541, y=u32 2 ("milliseconds to wait")) -> (x = y?=w539:bool)
        n333 = Select(t=T24."Disabled and Grayed Out" ("Disabled"), s=w539, f=T24."Enabled" ("Disabled")) -> (s? t:f=w536:T24)
        n334 = property on="Compression" class="Slide (strict)"("DisabledEnum"=w536) -> ()  [unwired: 2 in, 2 out]
      }
      event "Tree": Double Click {
        n335 = event-data() -> ("PlatMods"=w546:T27, "Tag"=w545:string)  [unwired: 1 in]
        n336 = Unbundle(w546) -> ("Shift"=w544:bool)  [unwired: 4 out]
        n337 = Not(x=w544) -> (.not. x?=w543:bool)
        n338 = call <vilib>:"NT Update Persistence.vi"("Persistence"=w543, "Name"=w545) -> ()  [unwired: 9 in, 1 out]
      }
    }
  }
  n339 = while {
    tunnel: w47 -> [w550]
    i -> [w553]
    stop <- FALSE stop-if-true
    n340 = Wait (ms)(milliseconds to wait=u32 100) -> ()  [unwired: 1 out]
    n341 = case shown="\"Playback\"" "Rec Mode" {
      tunnel: w553 -> [_ _ w568]
      tunnel: [u32 2829099 ("Base Color") u32 11141120 ("Target Color") w557] -> w549
      frame "Stop", Default {
        # "Reset the color, extra updates don't cost much"
      }
      frame "Record" {
      }
      frame "Playback" {
        # "Playback"
        n342 = Quotient & Remainder(x=w568, y=u32 50 ("milliseconds to wait")) -> (x-y*floor(x/y)=w564:u32)  [unwired: 1 out]
        n343 = Divide(x=w564, y=u32 50 ("milliseconds to wait")) -> (x/y=w561:dbl)
        n344 = Multiply(x=6.283185307179586, y=w561) -> (x*y=w566:dbl)
        n345 = Sine(x=w566) -> (sin(x)=w565:dbl)
        n346 = Absolute Value(x=w565) -> (abs(x)=w558:dbl)
        n347 = call "Interpolate RGB Color.vi"("Proportion"=w558, "Target Color"=u32 30976, "Base Color"=u32 2829099) -> ("Result Color"=w557:u32)  [unwired: 8 in]
      }
    }
    n348 = property class="Pane"(reference=w550, "PaneColor"=w549) -> ()  [unwired: 1 in, 2 out]
  }
  n349 = local write "Dashboard Tab"(T1."Drive" ("Dashboard Tab")) -> ()
  n350 = property on="On/Off" class="Bool (strict)"("Visible"=w15) -> ()  [unwired: 2 in, 2 out]
  n351 = property on="Motor" class="Clust (strict)"("Visible"=w15) -> ()  [unwired: 2 in, 2 out]
  n352 = property on="Progress" class="Clust (strict)"("Visible"=w15) -> ()  [unwired: 2 in, 2 out]
  n353 = property on="Test Ring" class="Ring (strict)"("Visible"=w15) -> ()  [unwired: 2 in, 2 out]
  n354 = property on="Rev/Fwd" class="Clust (strict)"("Visible"=w15) -> ()  [unwired: 2 in, 2 out]
  n355 = property on="Camera Settings" class="Clust (strict)"("Visible"=w15) -> ()  [unwired: 2 in, 2 out]
  n356 = local write "DB Camera Config"(w15) -> ()
  n357 = local write "Command Params"(string[][] [] ("Command Params")) -> ()
  n358 = global write "WPI_DashboardLogging Global.vi" "Recording"(w41) -> ()
  n359 = local write "Rec Mode"(w41) -> ()
  n360 = while {
    tunnel: u16 1741 ("timeout ms (25000)") -> [w570]
    stop <- FALSE stop-if-true
    n361 = TCP Create Listener(10:w570) -> (0:w569:errorcluster, 3:w571:refnum<k5>)  [unwired: 4 in, 1 out]
    n362 = case shown="No Error" w569 {
      selector: w569 -> [w573 _]
      tunnel: w571 -> [w574 _]
      frame No Error {
        n363 = while {
          tunnel: w574 -> [w577]
          tunnel: w573 -> [w576]
          stop <- FALSE stop-if-true
          n364 = TCP Wait On Listener(8:w576, 11:w577) -> (0:w578:errorcluster, 4:w579:refnum<k5>)  [unwired: 2 in, 3 out]
          n365 = local write "TCP"(w579) -> ()
          n366 = case shown="No Error" w578 {
            frame No Error {
            }
            frame Error {
              n367 = Wait (ms)(milliseconds to wait=u32 1000) -> ()  [unwired: 1 out]
            }
          }
        }
      }
      frame Error {
        n368 = Wait (ms)(milliseconds to wait=u32 1000) -> ()  [unwired: 1 out]
      }
    }
  }
  n369 = local write "Command Selection"(u16 0 ("milliseconds to wait")) -> ()
